vi "Example - Single Measurement.vi"() -> ()   [LabVIEW 2012]
panel:
  in  "Location of FieldMax2Lib.dll in":path=path "C:/Windows/System32/FieldMax2Lib.dll"
  out "Meter Serial Number":string
  out "Measurement":sgl
  # "This example for collecting data just returns a single measurement value instead of streaming measurements.  The VI will automatically stop after the first valid measurement is collected.  This can be useful if measurements are being taken on an interval instead of every data point being collected."
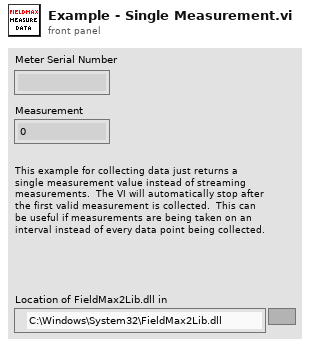
[diagram p1: front panel]
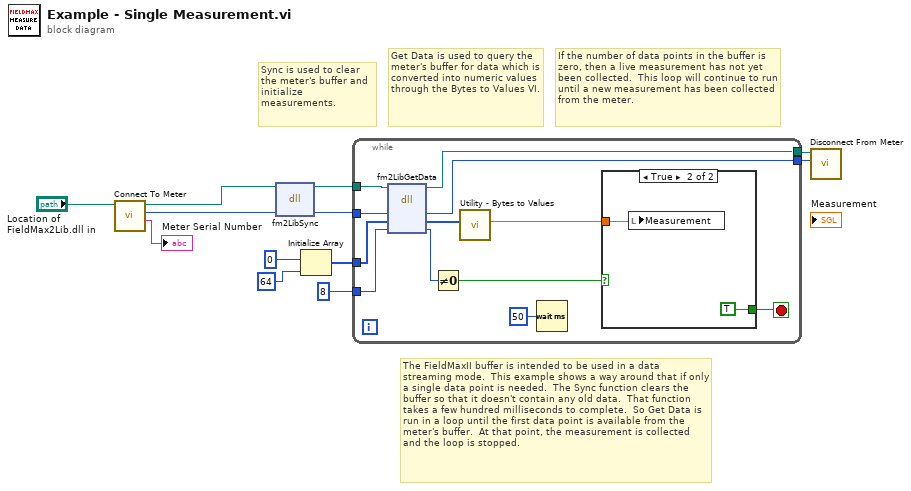
[diagram p0: block diagram]
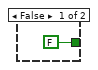
[diagram p2: hidden frame]
diagram:
  # "The FieldMaxII buffer is intended to be used in a data streaming mode.  This example shows a way around that if only a single data point is needed.  The Sync function clears the buffer so that it doesn't contain any old data.  That function takes a few hundred milliseconds to complete.  So Get Data is run in a loop until the first data point is available from the meter's buffer.  At that point, the measurement is collected and the loop is stopped."
  # "If the number of data points in the buffer is zero, then a live measurement has not yet been collected.  This loop will continue to run until a new measurement has been collected from the meter."
  # "Get Data is used to query the meter's buffer for data which is converted into numeric values through the Bytes to Values VI."
  # "Sync is used to clear the meter's buffer and initialize measurements."
  n1 = call "Connect To Meter.vi"("Location of FieldMax2Lib.dll in"="Location of FieldMax2Lib.dll in") -> ("Meter Serial Number"=→"Meter Serial Number":string, "Meter ID out"=w3:i32, "Location of FieldMax2Lib.dll out"=w4:path)  [unwired: 6 in]
  n2 = dll-call lib="C:/Windows/System32/FieldMax2Lib.dll" fn="fm2LibSync" label="Sync"(path in=w4, "h"=w3) -> (path out=w2:path, "h"=w1:i32)  [unwired: 3 in, 1 out]
  n3 = Initialize Array(u8 0 ("element"), 64 ("dimension size")) -> (w10:u8[])
  n4 = while {
    tunnel: w1 -> [w14]
    tunnel: w10 -> [w20]
    tunnel: i16 8 ("count") -> [w19]
    tunnel: [w16] -> w6
    tunnel: w2 -> [w21]
    tunnel: [w15] -> w5
    stop <- w13 stop-if-true
    n5 = dll-call lib="C:/Windows/System32/FieldMax2Lib.dll" fn="fm2LibGetData" label="Get Data"(path in=w21, "h"=w14, "returnBuffer"=w20, "count"=w19) -> (path out=w15:path, "h"=w16:i32, "returnBuffer"=w17:u8[], "count"=w18:i16)  [unwired: 3 in, 1 out]
    n6 = Not Equal To 0?(x=w18) -> (x != 0?=w22:bool)
    n7 = call "Utility - Bytes to Values.vi"("DataBuffer"=w17) -> ("Measurement Value"=w23:sgl)  [unwired: 9 in, 1 out]
    n8 = Wait (ms)(milliseconds to wait=u32 50) -> ()  [unwired: 1 out]
    n9 = case shown="True" w22 {
      tunnel: w23 -> [_ w27]
      tunnel: [FALSE TRUE] -> w13
      frame False {
      }
      frame True {
        n10 = local write "Measurement"(w27) -> ()
      }
    }
  }
  n11 = call "Disconnect From Meter.vi"("Location of FieldMax2Lib.dll in"=w5, "Meter ID in"=w6) -> ()  [unwired: 7 in, 2 out]
